vi "test_cs.vi"() -> ()   [LabVIEW 2013]
uses:
  lightfield-automation-labview/VIs/ClientServerMode/CS_LFAClassGlobal.vi
  lightfield-automation-labview/LightField Automation.lvclass
panel:
  in  "Delete File?":bool
  in  "Capture Frames":i32=-1
  in  "Capture":bool
  out "Capture ROI 1, Frame 1, Row 2":dbl[](graph)
  out "Acquire ROI 1, Frame 1, Row 1":dbl[](graph)
  in  "Acquire":bool
  out "Capture ROI 1, Frame 1":dbl[][](graph)
  out "Acquire ROI 1, Frame 1":dbl[][](graph)
  in  "?":bool
  out "Exposures Per Frame":i32
  in  "Exposures Per Frame":i32=1
  out "Number of Frames":i32
  in  "Number of Frames":i32=1
  out "Exposure Time (s)":dbl
  in  "Exposure Time (s)":dbl=0.1
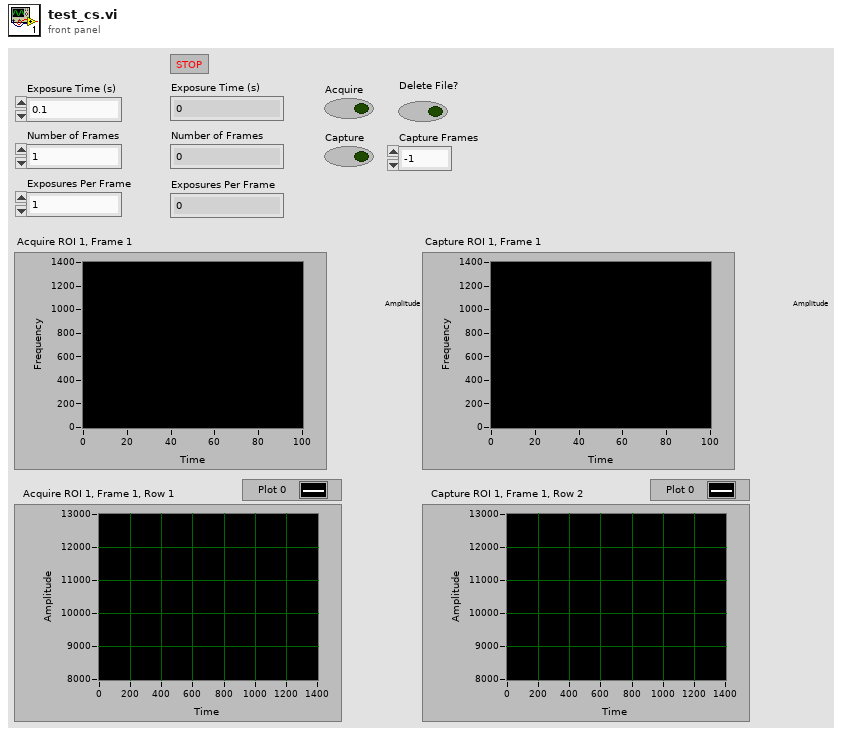
[diagram p1: front panel]
types:
  T1 = cluster{"Image":dbl[][][], "Frame Size":cluster{"F":i32, "Y":i32, "X":i32}}[]
  T2 = cluster{"Image":dbl[][][], "Frame Size":cluster{"F":i32, "Y":i32, "X":i32}}
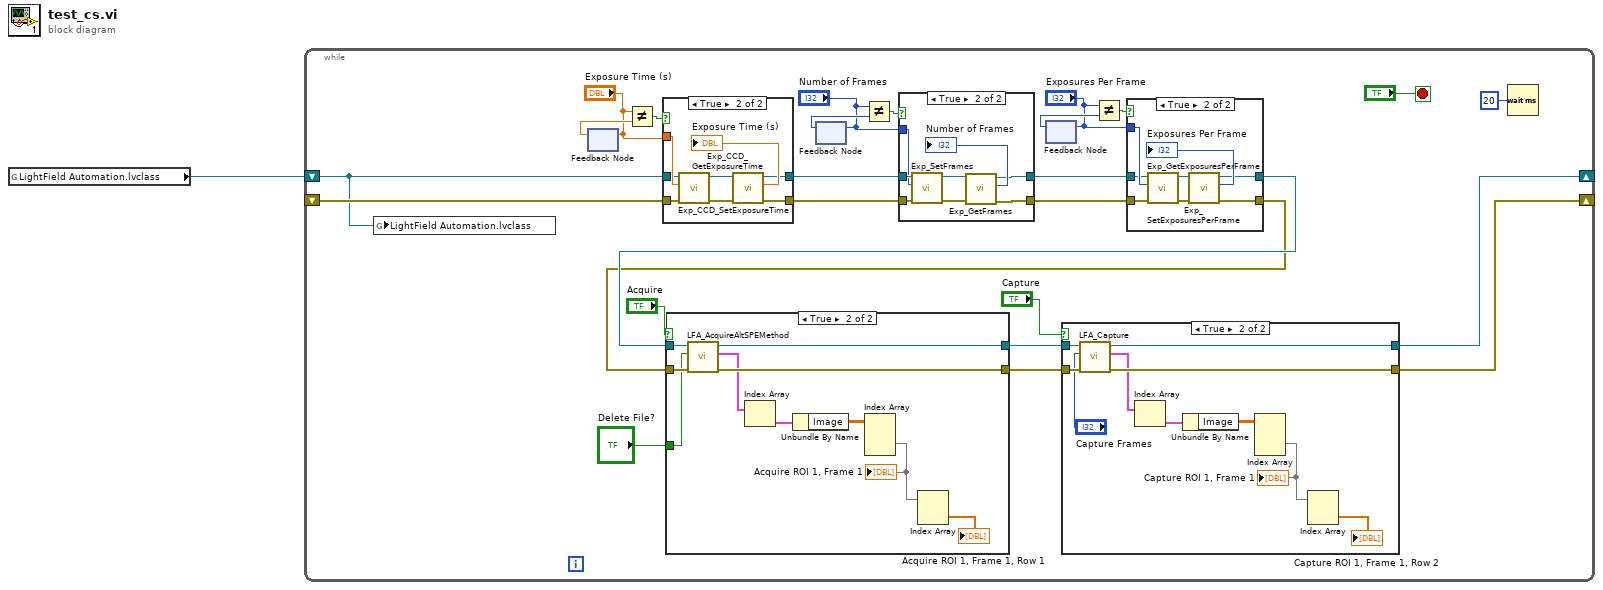
[diagram p0: block diagram]
diagram:
  n1 = global read "CS_LFAClassGlobal.vi" "LightField Automation.lvclass"() -> (w1:refnum<class "LightField Automation.lvclass">)
  n2 = while {
    shift-right: [w7] -> _
    shift-left: w1 -> [w2]
    shift-right: [w6] -> _
    shift-left: _ -> [w3]
    stop <- "?" stop-if-true
    n3 = global write "CS_LFAClassGlobal.vi" "LightField Automation.lvclass"(w2) -> ()
    n4 = feedback-in #1("Exposure Time (s)") -> ()
    n5 = feedback #1() -> (w24:dbl)  [unwired: 1 in]
    n6 = Not Equal?(x="Exposure Time (s)", y=w24) -> (x != y?=w25:bool)
    n7 = case shown="True" w25 {
      tunnel: "Exposure Time (s)" -> [_ w78]
      tunnel: w2 -> [w72 w77]
      tunnel: w3 -> [w73 w76]
      tunnel: [w72 w75] -> w22
      tunnel: [w73 w74] -> w21
      frame False {
      }
      frame True {
        n8 = call "Exp_CCD_SetExposureTime.vi"("error in (no error)"=w76, "Exposure Time (s)"=w78, "LightField Automation in"=w77) -> ("error out"=w79:errorcluster, "LightField Automation out"=w80:refnum<class "LightField Automation.lvclass">)  [unwired: 7 in]
        n9 = call "Exp_CCD_GetExposureTime.vi"("error in (no error)"=w79, "LightField Automation in"=w80) -> ("error out"=w74:errorcluster, "Exposure Time (s)"=→"Exposure Time (s)":dbl, "LightField Automation out"=w75:refnum<class "LightField Automation.lvclass">)  [unwired: 7 in]
      }
    }
    n10 = feedback #2() -> (w20:i32)  [unwired: 1 in]
    n11 = feedback-in #2("Number of Frames") -> ()
    n12 = Not Equal?(x="Number of Frames", y=w20) -> (x != y?=w19:bool)
    n13 = case shown="True" w19 {
      tunnel: w22 -> [w63 w68]
      tunnel: w21 -> [w62 w67]
      tunnel: "Number of Frames" -> [_ w66]
      tunnel: [w63 w65] -> w14
      tunnel: [w62 w64] -> w13
      frame False {
      }
      frame True {
        n14 = call "Exp_SetFrames.vi"("error in (no error)"=w67, "Number of Frames"=w66, "LightField Automation in"=w68) -> ("error out"=w70:errorcluster, "LightField Automation out"=w71:refnum<class "LightField Automation.lvclass">)  [unwired: 7 in]
        n15 = call "Exp_GetFrames.vi"("error in (no error)"=w70, "LightField Automation in"=w71) -> ("error out"=w64:errorcluster, "Frames"=→"Number of Frames":i32, "LightField Automation out"=w65:refnum<class "LightField Automation.lvclass">)  [unwired: 7 in]
      }
    }
    n16 = feedback #3() -> (w17:i32)  [unwired: 1 in]
    n17 = feedback-in #3("Exposures Per Frame") -> ()
    n18 = Not Equal?(x="Exposures Per Frame", y=w17) -> (x != y?=w16:bool)
    n19 = case shown="True" w16 {
      tunnel: "Exposures Per Frame" -> [_ w58]
      tunnel: w14 -> [w53 w57]
      tunnel: w13 -> [w52 w56]
      tunnel: [w52 w55] -> w10
      tunnel: [w53 w54] -> w12
      frame False {
      }
      frame True {
        n20 = call "Exp_SetExposuresPerFrame.vi"("error in (no error)"=w56, "Exposures Per Frame"=w58, "LightField Automation in"=w57) -> ("error out"=w61:errorcluster, "LightField Automation out"=w60:refnum<class "LightField Automation.lvclass">)  [unwired: 7 in]
        n21 = call "Exp_GetExposuresPerFrame.vi"("error in (no error)"=w61, "LightField Automation in"=w60) -> ("error out"=w55:errorcluster, "Exposures Per Frame"=→"Exposures Per Frame":i32, "LightField Automation out"=w54:refnum<class "LightField Automation.lvclass">)  [unwired: 7 in]
      }
    }
    n22 = case shown="True" "Acquire" {
      tunnel: w12 -> [w41 w47]
      tunnel: w10 -> [w40 w46]
      tunnel: [w41 w44] -> w9
      tunnel: [w40 w43] -> w8
      tunnel: "Delete File?" -> [_ w45]
      frame False {
      }
      frame True {
        n23 = call "LFA_AcquireAltSPEMethod.vi"("error in (no error)"=w46, "Delete File?"=w45, "LightField Automation in"=w47) -> ("error out"=w43:errorcluster, "Data"=w42:T1, "LightField Automation out"=w44:refnum<class "LightField Automation.lvclass">)  [unwired: 6 in]
        n24 = Index Array(array=w42) -> (element=w51:T2)  [unwired: 1 in]
        n25 = Unbundle By Name(w51) -> ("Image"=w50:dbl[][][])
        n26 = Index Array(array=w50) -> (element=w49:dbl[][])  [unwired: 3 in]
        "Acquire ROI 1, Frame 1" <- w49
        n27 = Index Array(array=w49) -> (element=→"Acquire ROI 1, Frame 1, Row 1":dbl[])  [unwired: 2 in]
      }
    }
    n28 = case shown="True" "Capture" {
      tunnel: w9 -> [w29 w35]
      tunnel: w8 -> [w28 w34]
      tunnel: [w29 w32] -> w7
      tunnel: [w28 w33] -> w6
      frame False {
      }
      frame True {
        n29 = call "LFA_Capture.vi"("error in (no error)"=w34, "Frames"="Capture Frames", "LightField Automation in"=w35) -> ("error out"=w33:errorcluster, "Data"=w31:T1, "LightField Automation out"=w32:refnum<class "LightField Automation.lvclass">)  [unwired: 6 in]
        n30 = Index Array(array=w31) -> (element=w39:T2)  [unwired: 1 in]
        n31 = Unbundle By Name(w39) -> ("Image"=w38:dbl[][][])
        n32 = Index Array(array=w38) -> (element=w36:dbl[][])  [unwired: 3 in]
        "Capture ROI 1, Frame 1" <- w36
        n33 = Index Array(array=w36) -> (element=→"Capture ROI 1, Frame 1, Row 2":dbl[])  [unwired: 2 in]
      }
    }
    n34 = Wait (ms)(milliseconds to wait=u32 20) -> ()  [unwired: 1 out]
  }
